vi "Obtain Notifier.vi"(8 "error in (no error)":errorcluster, 11 "CVT_I32 in":refnum<class "CVT_I32.lvclass">) -> (0 "error out":errorcluster, 3 "CVT_I32 out":refnum<class "CVT_I32.lvclass">)   [LabVIEW 2024, in "Current Value Table.lvlib" / "CVT_I32.lvclass"]
uses:
  CVT_I32.lvclass
  CVT_I32.lvclass/CVT_I32.ctl
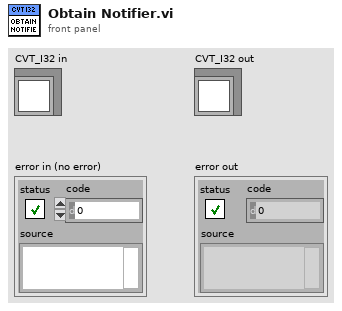
[diagram p1: front panel]
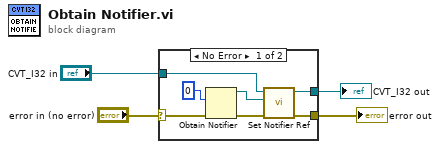
[diagram p0: block diagram]
diagram:
  n1 = case shown="No Error" "error in (no error)" {
    selector: "error in (no error)" -> [w11 w13]
    tunnel: [w6 w13] -> w3
    tunnel: [w9 w12] -> w1
    tunnel: "CVT_I32 in" -> [w10 w12]
    frame No Error {
      n2 = Obtain Notifier(notification data type=0 ("element data type"), error in (no error)=w11) -> (notifier out=w8:refnum<notifier>, error out=w7:errorcluster)  [unwired: 2 in, 1 out]
      n3 = call-dynamic "Set Notifier Ref.vi"("error in (no error)"=w7, "notifier in"=w8, "CVT_I32 in"=w10) -> ("error out"=w6:errorcluster, "CVT_I32 out"=w9:refnum<class "CVT_I32.lvclass">)  [unwired: 7 in]
    }
    frame Error {
    }
  }
  "error out" <- w3
  "CVT_I32 out" <- w1
